vi "pico_ctlstostring_2.vi"(1 "Response?":bool, 2 "AXIS":u16(ring) items=["X", "Y or SLIDE", "Z"], 3 "MIRRORS":u16=1, 4 "aRate":dbl=1370.408163265306 format="%.2f", 5 "ARateButton":bool, 6 "aDir":bool=TRUE, 7 "aStop":bool, 8 "APulses":u16=300, 9 "APulsesButton":bool) -> (0 "String out":string)   [LabVIEW 2013]
panel:
  # "Picomotor Controls to String"
  # "This VI parses pico control values into a string  for TCP transmission"
  # "The strings generated are:\nstop\nrate:XXXX  sets the rate to XXXX\ngo:XXXX:dir:chan:axis  where dir=cw or ccw, chan and axis are integers \n                                      moves chan,axis by XXXX in direction dir"
  # "Target Rate"
  # "Pulse RATE"
  # "Do # PULSES"
  # "DIRECTION"
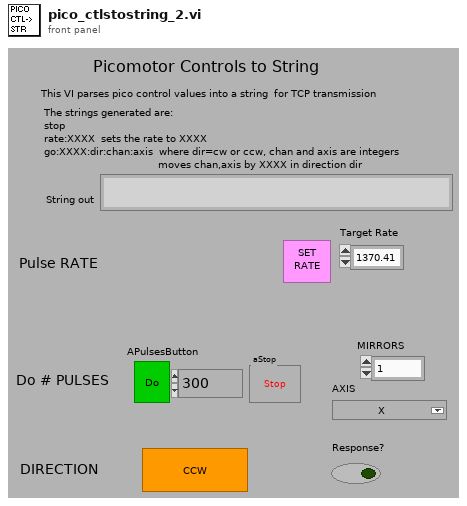
[diagram p1: front panel]
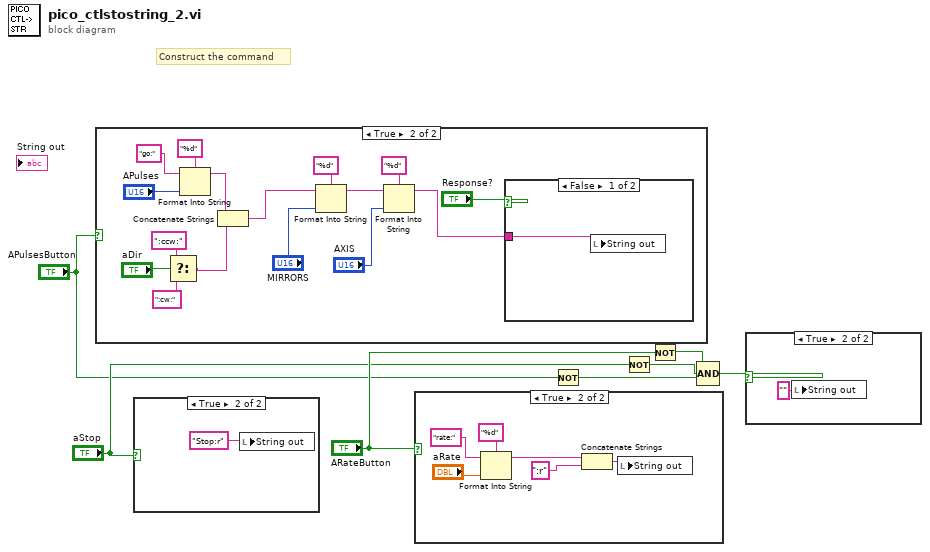
[diagram p0: block diagram]
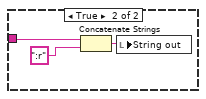
[diagram p6: hidden frame]
diagram:
  # "Construct the command"
  n1 = case shown="True" "APulsesButton" {
    frame False {
    }
    frame True {
      n2 = Select(t=":ccw:", s="aDir", f=":cw:") -> (s? t:f=w15:string)
      n3 = Format Into String(format string="%d", initial string="go:", "APulses") -> (resulting string=w16:string)  [unwired: 1 in, 1 out]
      n4 = Concatenate Strings(w16, w15) -> (w14:string)
      n5 = Format Into String(format string="%d", initial string=w14, "MIRRORS") -> (resulting string=w9:string)  [unwired: 1 in, 1 out]
      n6 = Format Into String(format string="%d", initial string=w9, "AXIS") -> (resulting string=w8:string)  [unwired: 1 in, 1 out]
      n7 = case shown="False" "Response?" {
        tunnel: w8 -> [w24 w26]
        frame False {
          n8 = local write "String out"(w24) -> ()
        }
        frame True {
          n9 = Concatenate Strings(w26, ":r" ("string")) -> (w25:string)
          n10 = local write "String out"(w25) -> ()
        }
      }
    }
  }
  n11 = case shown="True" "aStop" {
    frame False {
    }
    frame True {
      n12 = local write "String out"("Stop:r" ("String out")) -> ()
    }
  }
  n13 = case shown="True" "ARateButton" {
    frame False {
    }
    frame True {
      n14 = Format Into String(format string="%d", initial string="rate:", "aRate") -> (resulting string=w30:string)  [unwired: 1 in, 1 out]
      n15 = Concatenate Strings(w30, ":r" ("string")) -> (w31:string)
      n16 = local write "String out"(w31) -> ()
    }
  }
  n17 = Not(x="APulsesButton") -> (.not. x?=w4:bool)
  n18 = Not(x="aStop") -> (.not. x?=w3:bool)
  n19 = Not(x="ARateButton") -> (.not. x?=w2:bool)
  n20 = Compound Arithmetic op=AND ("And")(w2, w3, w4) -> (w1:bool)
  n21 = case shown="True" w1 {
    frame False {
    }
    frame True {
      n22 = local write "String out"("" ("String out")) -> ()
    }
  }
